vi "Close.vi"(8 "error in":errorcluster, 11 "Temperature Setpoint in":refnum<class "Temperature Setpoint.lvclass">) -> (0 "error out":errorcluster, 3 "Temperature Setpoint out":refnum<class "Temperature Setpoint.lvclass">)   [LabVIEW 2023, in "Temperature Setpoint.lvclass"]
uses:
  Temperature Setpoint.lvclass
  Temperature Setpoint.lvclass/Temperature Setpoint.ctl
  Parents/Setpoint/Setpoint.lvclass
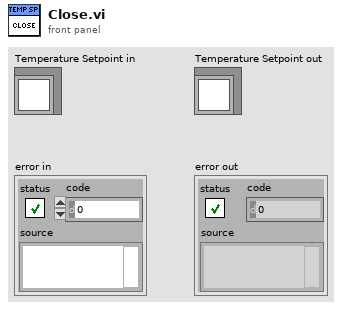
[diagram p1: front panel]
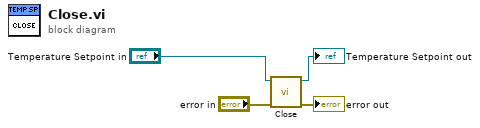
[diagram p0: block diagram]
diagram:
  n1 = call-parent "Close.vi"("error in"="error in", "Setpoint in"="Temperature Setpoint in") -> ("error out"=→"error out":errorcluster, "Setpoint out"=→"Temperature Setpoint out":refnum<class "Temperature Setpoint.lvclass">)  [unwired: 8 in]
